vi "Actor Core.vi"(8 "error in":errorcluster, 11 "Humidifier in":refnum<class "Humidifier.lvclass">) -> (0 "error out":errorcluster, 3 "Actor out":refnum<class "Actor.lvclass">)   [LabVIEW 2014, in "Humidifier Lib.lvlib" / "Humidifier.lvclass"]
doc: "(<B>Filename</B>: Actor Framework.lvlib:Actor.lvclass:Actor Core.vi)\n\nReceives messages to the actor, reacts to them, and initiates any error handling that may shut the actor down.\n\nDescendant classes may override this VI to append parallel tasks for the actor to complete while it handles messages. Overrides use the Call Parent Method node."
uses:
  Humidifier.lvclass
  <vilib>/ActorFramework/Actor/Actor.lvclass
  Humidifier.lvclass/Humidifier.ctl
  reusable/Command/Command.lvclass
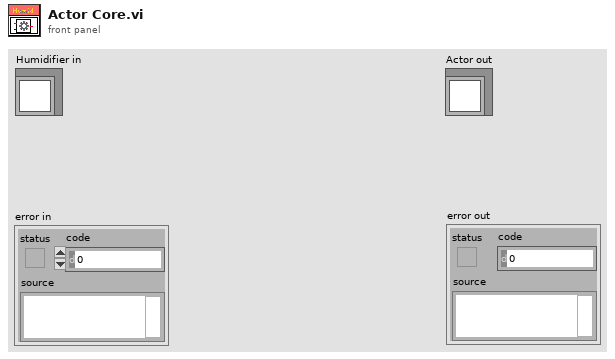
[diagram p1: front panel]
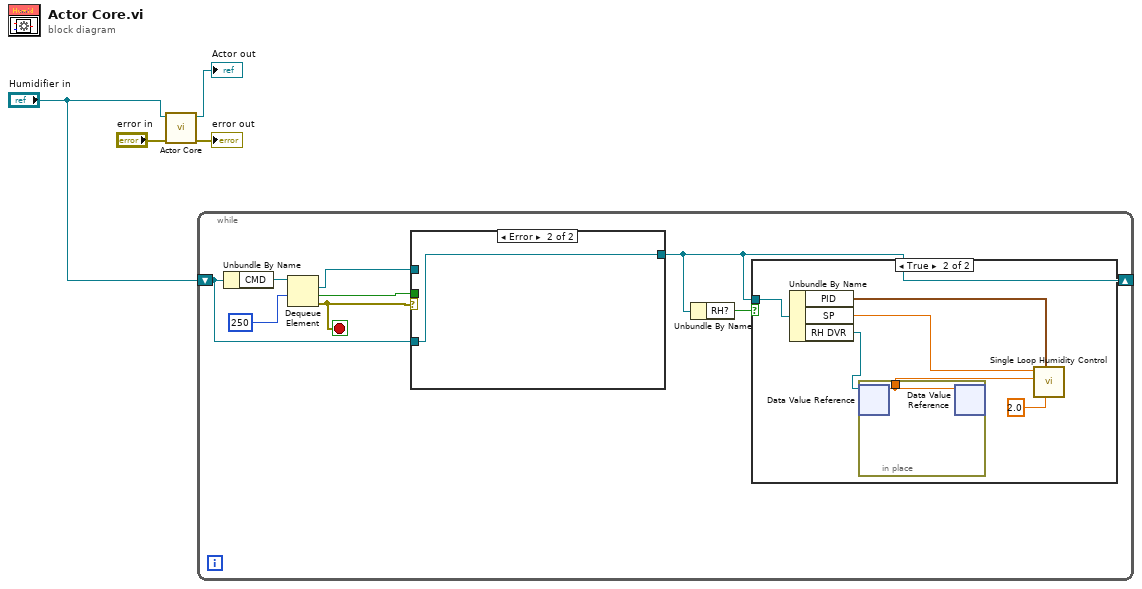
[diagram p0: block diagram]
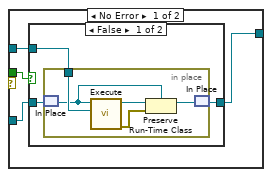
[diagram p3: hidden frame]
diagram:
  n1 = call-parent "Actor Core.vi"("error in"="error in", "Actor in"="Humidifier in") -> ("error out"=→"error out":errorcluster, "Actor out"=→"Actor out":refnum<class "Actor.lvclass">)  [unwired: 8 in]
  n2 = while {
    shift-right: [w5] -> _
    shift-left: "Humidifier in" -> [w7]
    stop <- w10 stop-if-true
    n3 = Unbundle By Name(w7) -> ("CMD"=w12:refnum<queue>)
    n4 = Dequeue Element(queue=w12, timeout in ms (-1)=250) -> (element=w8:refnum<class "Command.lvclass">, timed out?=w9:bool, error out=w10:errorcluster)  [unwired: 1 in, 1 out]
    n5 = case shown="Error" w10 {
      tunnel: w9 -> [w23 _]
      tunnel: w8 -> [w22 _]
      tunnel: w7 -> [w21 w33]
      tunnel: [w20 w33] -> w5
      frame No Error {
        n6 = case shown="False" w23 {
          tunnel: w21 -> [w26 w32]
          tunnel: [w25 w32] -> w20
          tunnel: w22 -> [w24 _]
          frame False {
            n7 = in-place {
              in-place-border: w24 -> [w31]
              n8 = in-place-match #1(w26) -> (w30:refnum<class "Humidifier.lvclass">)
              n9 = call-dynamic "Execute.vi"("Command in"=w31, "Object In"=w30) -> ("error out"=w27:errorcluster, "Object Out"=w29:refnum<class>)  [unwired: 8 in]
              n10 = Preserve Run-Time Class(object in=w29, error in=w27, 2:w30) -> (object out=w28:refnum<class "Humidifier.lvclass">)  [unwired: 1 out]
              n11 = in-place-match #1(w28) -> (w25:refnum<class "Humidifier.lvclass">)
            }
          }
          frame True {
          }
        }
      }
      frame Error {
      }
    }
    n12 = Unbundle By Name(w5) -> ("RH?"=w6:bool)
    n13 = case shown="True" w6 {
      tunnel: w5 -> [_ w18]
      frame False {
      }
      frame True {
        n14 = Unbundle By Name(w18) -> ("PID"=w17:cluster{"P":sgl, "I":sgl, "D":sgl}, "SP"=w16:sgl, "RH DVR"=w15:refnum<data-value>)
        n15 = in-place {
          in-place-border: [w19] -> w14
          n16 = in-place-dvr #2(w15) -> (w19:sgl)  [unwired: 1 out]
          n17 = in-place-dvr #2(w19) -> ()  [unwired: 2 out]
        }
        n18 = call "Single Loop Humidity Control.vi"("dt (s)"=2.0, "PID gains"=w17, "RHmeas"=w14, "RHsp"=w16) -> ()  [unwired: 6 in, 2 out]
      }
    }
  }
